vi "Single Pole IIR Filter Reset - fxp 20_3.vi"(0 "reset cycles-1":fxp<+,6,6>, 1 "reset":bool) -> (4 "reset done":bool, 6 "reset out":bool)   [LabVIEW 2017, in "FlexRIO ADC v1.lvlib"]
uses:
  <instrlib>/FlexRIO/API/FPGA/v1/IP/ADC/FlexRIO ADC v1.lvlib
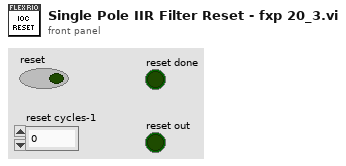
[diagram p1: front panel]
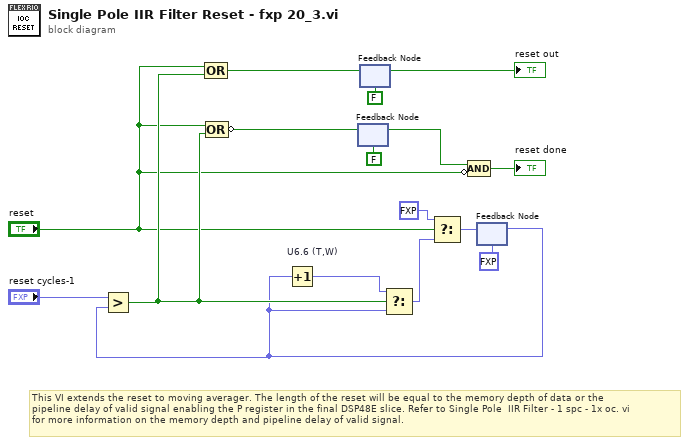
[diagram p0: block diagram]
diagram:
  # "This VI extends the reset to moving averager. The length of the reset will be equal to the memory depth of data or the \npipeline delay of valid signal enabling the P register in the final DSP48E slice. Refer to Single Pole  IIR Filter - 1 spc - 1x oc. vi \nfor more information on the memory depth and pipeline delay of valid signal."
  n1 = feedback #1(FALSE) -> (w2:bool)
  n2 = feedback #2(FALSE) -> (→"reset out":bool)
  n3 = Compound Arithmetic op=AND(w2, invert "reset") -> (→"reset done":bool)
  n4 = feedback #3(fxp<+,6,6> 0.0 ("period")) -> (w7:fxp<+,6,6>)
  n5 = Greater?(x="reset cycles-1", y=w7) -> (0:w10:bool)
  n6 = Compound Arithmetic op=OR("reset", w10) -> (w11:bool)
  n7 = Compound Arithmetic op=OR("reset", w10) -> (invert w9:bool)
  n8 = Increment "U6.6 (T,W)"(x=w7) -> (x+1=w8:fxp<+,6,6>)
  n9 = feedback-in #1(w9) -> ()
  n10 = feedback-in #2(w11) -> ()
  n11 = Select(t=w8, s=w10, f=w7) -> (s? t:f=w15:fxp<+,6,6>)
  n12 = Select(t=fxp<+,6,6> 0.0 ("period"), s="reset", f=w15) -> (s? t:f=w14:fxp<+,6,6>)
  n13 = feedback-in #3(w14) -> ()
